vi "CVT2GroupNamesTest.vi"() -> (3 "Unit Test Framework Results":T1)   [LabVIEW 2013, in "UnitTests.lvlib"]
uses:
  UnitTests.lvlib
  <vilib>/utf/common/utf_test_result_troll.ctl
  <vilib>/utf/common/utf_test_result.ctl
  <vilib>/utf/common/utf_test_result_failure.ctl
  <vilib>/utf/common/utf_test_comparison_operators.ctl
  <vilib>/utf/common/utf_vi_tag.ctl
  <vilib>/NI/Current Value Table/FGVs/Group Memory.vi
  <vilib>/utf/NI_UnitTestFramework.lvlib
  <vilib>/NI/Current Value Table/Current Value Table.lvlib
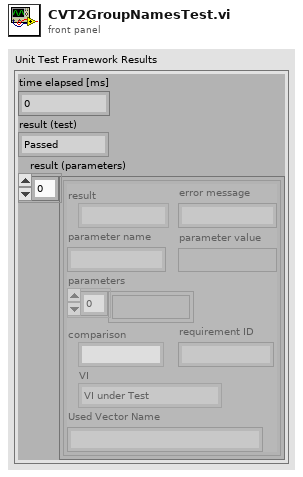
[diagram p1: front panel]
types:
  T1 = typedef "NI_UnitTestFramework.lvlib/utf_test_result_troll.ctl" = cluster{"time elapsed [ms]":u32, "result (test)":T2, "result (parameters)":T3[]}
  T2 = typedef "NI_UnitTestFramework.lvlib/utf_test_result.ctl" = enum16{"Passed", "Failed", "Error", "Skipped", "Not Processed"}
  T3 = typedef "NI_UnitTestFramework.lvlib/utf_test_result_failure.ctl" = cluster{"result":T2, "error message":string, "parameter name":string, "parameter value":variant, "parameters":variant[], "comparison":T4, "requirement ID":string, "VI":T5, "Used Vector Name":string}
  T4 = typedef "NI_UnitTestFramework.lvlib/utf_test_comparison_operators.ctl" = enum16{"=", "!=", ">", ">=", "<", "<=", "range", "symmetric tolerance", "asymmetric tolerance", "string contains", "string not contain", "array size", "string length", "array range", "by element", "array range (limit array)", "user-defined", "array contains", "array not contain", "vector length", "= (elm)", "!= (elm)", "= (case insensitive)", "!= (case insensitive)"}
  T5 = typedef "NI_UnitTestFramework.lvlib/utf_vi_tag.ctl" = enum16{"Setup VI", "VI under Test", "Teardown VI"}
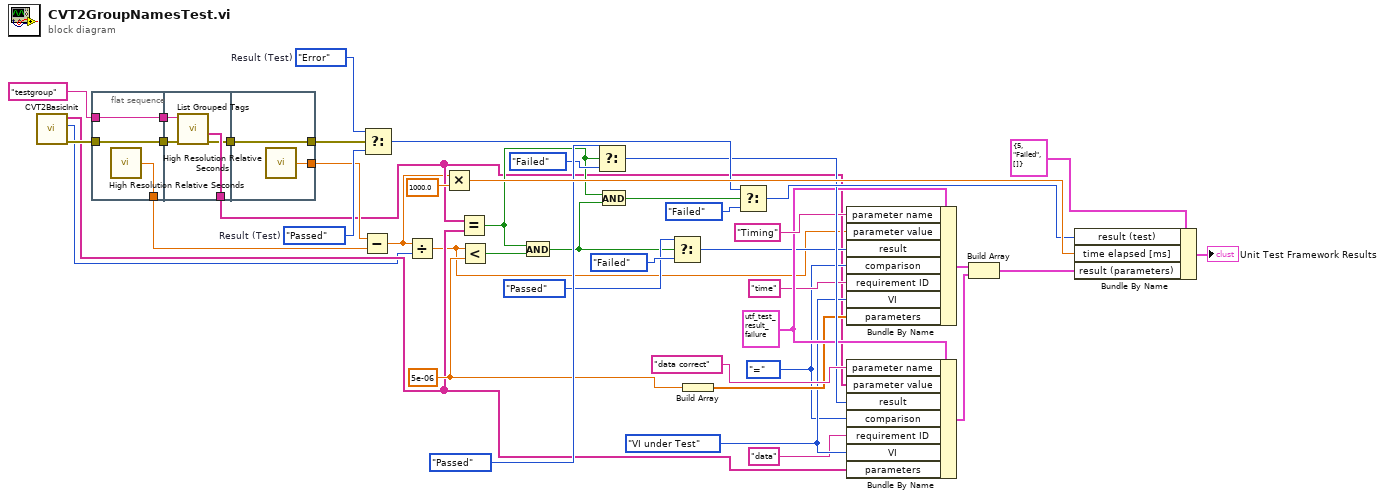
[diagram p0: block diagram]
diagram:
  w11 = 5e-06 ("y")
  w26 = T3 {"result"=enum."Passed", "error message"="", "parameter name"="", "parameter value"=variant, "parameters"=[], "comparison"=enum."=", "requirement ID"="", "VI"=enum."Setup VI", "Used Vector Name"=""} ("Unit Test Framework - result (parameters)")
  w19 = utf_test_comparison_operators."=" ("comparison")
  w21 = utf_vi_tag."VI under Test" ("VI")
  w41 = utf_test_result."Error"  # Result (Test)
  w40 = utf_test_result."Passed"  # Result (Test)
  n1 = call "CVT2BasicInit.vi"() -> ("error out"=w18:errorcluster, "Tags per type out"=w4:i32, "names"=w5:string[])  [unwired: 9 in]
  n2 = flat-sequence {
    tunnel: w18 -> [w47]
    tunnel: [w47] -> w16
    tunnel: [w46] -> w14
    tunnel: [w45] -> w8
    tunnel: "testgroup" ("Group") -> [w45]
    tunnel: [w49] -> w17
    tunnel: w16 -> [w51]
    tunnel: w8 -> [w48]
    tunnel: [w50] -> w6
    tunnel: [w53] -> w1
    tunnel: w17 -> [w53]
    tunnel: [w52] -> w15
    frame #0 {
      n3 = call <vilib>:"High Resolution Relative Seconds.vi"() -> ("relative seconds"=w46:dbl)
    }
    frame #1 {
      n4 = call <vilib>:"List Grouped Tags.vi"("error in (no error)"=w51, "Group"=w48) -> ("error out"=w49:errorcluster, "Tags Out"=w50:string[])  [unwired: 8 in]
    }
    frame #2 {
      n5 = call <vilib>:"High Resolution Relative Seconds.vi"() -> ("relative seconds"=w52:dbl)
    }
  }
  n6 = Subtract(x=w15, y=w14) -> (x-y=w2:dbl)
  n7 = Select(t=w41, s=w1, f=w40) -> (s? t:f=w37:T2)
  n8 = Divide(x=w2, y=w4) -> (x/y=w3:dbl)
  n9 = Multiply(x=w2, y=1000.0) -> (x*y=w38:dbl)
  n10 = Equal?(x=w6, y=w5) -> (x = y?=w12:bool)
  n11 = Less?(x=w3, y=w11) -> (x < y?=w13:bool)
  n12 = And(x=w12, y=w13) -> (x .and. y?=w10:bool)
  n13 = Select(t=utf_test_result."Passed" ("result"), s=w12, f=utf_test_result."Failed" ("result")) -> (s? t:f=w34:T2)
  n14 = And(x=w12, y=w10) -> (x .and. y?=w29:bool)
  n15 = Select(t=utf_test_result."Passed" ("result"), s=w10, f=utf_test_result."Failed" ("result")) -> (s? t:f=w24:T2)
  n16 = Build Array(w11) -> (w22:dbl[])
  n17 = Select(t=w37, s=w29, f=utf_test_result."Failed") -> (s? t:f=w35:T2)
  n18 = Bundle By Name(cluster=w26, "parameter name"="Timing", "parameter value"=w3, "result"=w24, "comparison"=w19, "requirement ID"="time", "VI"=w21, "parameters"=w22) -> (w28:T3)
  n19 = Bundle By Name(cluster=w26, "parameter name"="data correct", "parameter value"=w6, "result"=w34, "comparison"=w19, "requirement ID"="data", "VI"=w21, "parameters"=w5) -> (w31:T3)
  n20 = Build Array(w28, w31) -> (w30:T3[])
  n21 = Bundle By Name(cluster=T1 {"time elapsed [ms]"=5, "result (test)"=enum."Failed", "result (parameters)"=[]} ("Unit Test Framework - Result"), "result (test)"=w35, "time elapsed [ms]"=w38, "result (parameters)"=w30) -> (→"Unit Test Framework Results":T1)
